vi "TCP Wait For Specific Response Dll.vi"(0 "TCP Connection In":refnum<k5>, 5 "Expected Type":T2=enum."NONE", 7 "Expected Subtype (none)":T1, 9 "Timeout (250 ms)":i32=250) -> (4 "TCP Connection Out":refnum<k5>, 6 "StatusIsFalse":i16)   [LabVIEW 2011]
uses:
  Controls/QCA NART Response Type.ctl
  Controls/QCA NART Response SubType.ctl
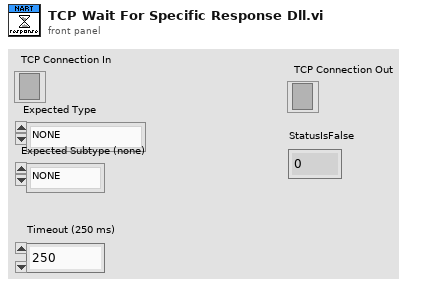
[diagram p1: front panel]
types:
  T1 = typedef "QCA NART Response SubType.ctl" = enum16{"NONE", "OK", "ON", "OFF", "BEGIN", "DONE"}
  T2 = typedef "QCA NART Response Type.ctl" = enum16{"DEBUG", "CONTROL", "INFO", "WARNING", "ERROR", "NONE"}
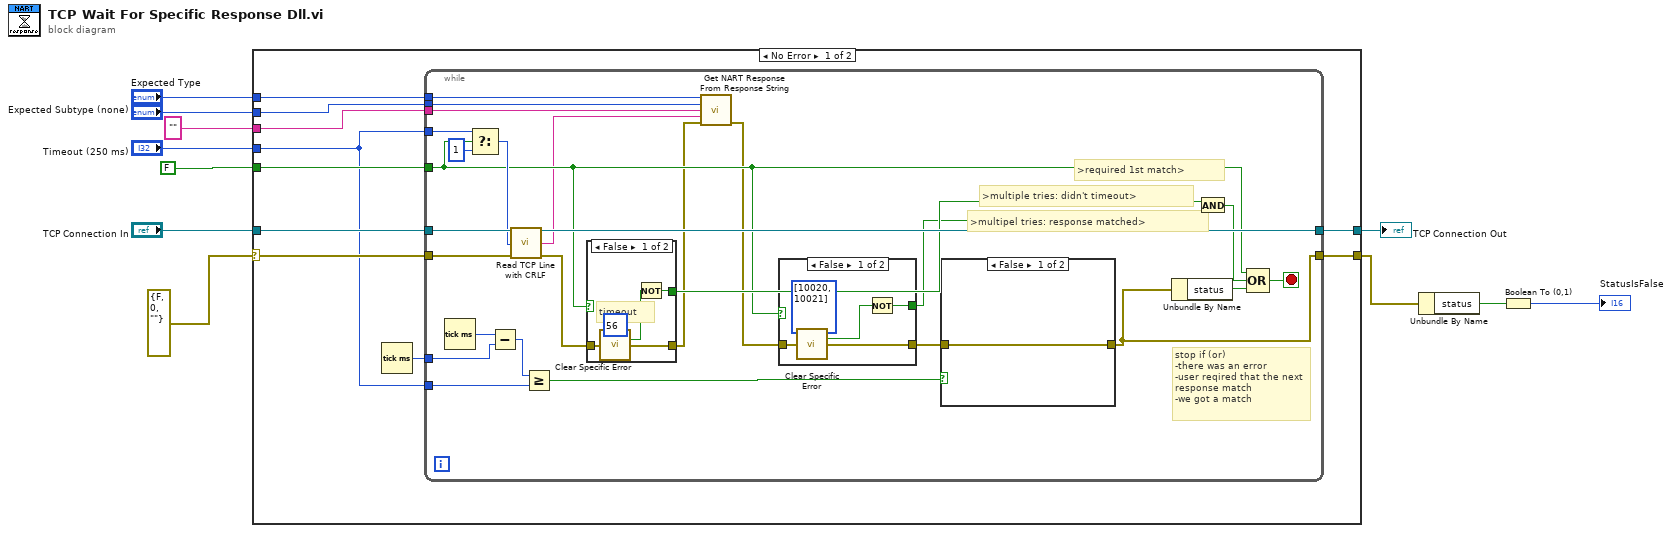
[diagram p0: block diagram]
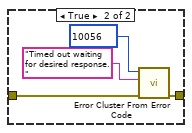
[diagram p4: hidden frame]
diagram:
  n1 = case shown="No Error" errorcluster {"status"=FALSE, "code"=0, "source"=""} ("error in") {
    selector: errorcluster {"status"=FALSE, "code"=0, "source"=""} ("error in") -> [w21 w66]
    tunnel: [w13 w66] -> w3
    tunnel: "TCP Connection In" -> [w20 w65]
    tunnel: [w19 w65] -> w10
    tunnel: "Timeout (250 ms)" -> [w14 _]
    tunnel: "Expected Type" -> [w18 _]
    tunnel: "Expected Subtype (none)" -> [w17 _]
    tunnel: FALSE ("Next response (f)") -> [w16 _]
    tunnel: "" ("Expected Message Start (\"\":any)") -> [w12 _]
    frame No Error {
      n2 = Tick Count (ms)() -> (millisecond timer value=w15:u32)
      n3 = while {
        tunnel: w21 -> [w47]
        tunnel: w20 -> [w46]
        tunnel: [w45] -> w19
        tunnel: w18 -> [w22]
        tunnel: w17 -> [w23]
        tunnel: w14 -> [w31]
        tunnel: w16 -> [w30]
        tunnel: w15 -> [w42]
        tunnel: w14 -> [w40]
        tunnel: [w36] -> w13
        tunnel: w12 -> [w24]
        stop <- w37 stop-if-true
        # ">required 1st match>"
        # ">multipel tries: response matched>"
        # ">multiple tries: didn't timeout>"
        # "stop if (or)\n-there was an error\n-user reqired that the next response match\n-we got a match"
        n4 = Tick Count (ms)() -> (millisecond timer value=w43:u32)
        n5 = Select(t=w31, s=w30, f=1) -> (s? t:f=w44:i32)
        n6 = Subtract(x=w43, y=w42) -> (x-y=w41:u32)
        n7 = call "Read TCP Line with CRLF.vi"("TCP Connection In"=w46, "timeout ms (100)"=w44, "error in"=w47) -> ("TCP Connection Out"=w45:refnum<k5>, "TCP Line"=w25:string, "error out"=w28:errorcluster)  [unwired: 10 in]
        n8 = Greater Or Equal?(x=w41, y=w40) -> (x >= y?=w39:bool)
        n9 = case shown="False" w30 {
          tunnel: w28 -> [w58 w59]
          tunnel: [w57 w59] -> w27
          tunnel: [w54 _] -> w34
          frame False {
            # "timeout"
            n10 = call "Clear Specific Error.vi"("Specific Error Number (0: none)"=56 ("Specific Error Number"), "error in"=w58) -> ("Error Cleared?"=w55:bool, "error out"=w57:errorcluster)  [unwired: 12 in]
            n11 = Not(x=w55) -> (.not. x?=w54:bool)
          }
          frame True {
            # "1 try"
          }
        }
        n12 = call "Get NART Response From Response String.vi"("Expected Response"=w22, "Response Subtype"=w23, "Expected Message start (\"\":any)"=w24, "TCP Line"=w25, "error in (no error)"=w27) -> ("error out"=w26:errorcluster)  [unwired: 9 in, 1 out]
        n13 = case shown="False" w30 {
          tunnel: w26 -> [w52 w53]
          tunnel: [w51 w53] -> w35
          tunnel: [w49 _] -> w33
          frame False {
            n14 = call "Clear Specific Error.vi"("Error Numbers Array (emtpy)"=i32[] [10020, 10021] ("Error Numbers Array"), "error in"=w52) -> ("Error Cleared?"=w50:bool, "error out"=w51:errorcluster)  [unwired: 12 in]
            n15 = Not(x=w50) -> (.not. x?=w49:bool)
          }
          frame True {
            # "1 try"
          }
        }
        n16 = case shown="False" w39 {
          tunnel: w35 -> [w60 w64]
          tunnel: [w60 w62] -> w36
          frame False {
          }
          frame True {
            n17 = call <vilib>:"Error Cluster From Error Code.vi"("error in (no error)"=w64, "error message (\"\")"="Timed out waiting for desired response." ("format string"), "error code (0)"=10056) -> ("error out"=w62:errorcluster)  [unwired: 6 in]
          }
        }
        n18 = Unbundle By Name(w36) -> ("status"=w38:bool)
        n19 = And(x=w34, y=w33) -> (x .and. y?=w32:bool)
        n20 = Compound Arithmetic op=OR(w30, w32, w38) -> (w37:bool)
      }
    }
    frame Error {
    }
  }
  "TCP Connection Out" <- w10
  n21 = Unbundle By Name(w3) -> ("status"=w2:bool)
  n22 = Boolean To (0,1)(Boolean=w2) -> (0, 1=→"StatusIsFalse":i16)
